vi "setFont.vi"(8 "Error In":errorcluster, 9 "className (\"QWidget\")":string="QWidget", 10 "font":refnum<class "QFont.lvclass">, 11 "LQWidgetEngine In":refnum<class "LQWidgetEngine.lvclass">) -> (0 "Error Out":errorcluster, 3 "LQWidgetEngine Out":refnum<class "LQWidgetEngine.lvclass">)   [LabVIEW 2014, in "LQWidgetEngine.lvclass"]
doc: "LabVIEW-specific documentation is not yet available. See <b>https://doc.qt.io/qt-5/qapplication.html#setFont</b>"
uses:
  LQWidgetEngine.lvclass
  Qt GUI/QFont/QFont.lvclass
  LQ Core/LQIdentity/LQIdentity.lvclass/LQIdentity.ctl
  LQ Core/LQSerialData/LQSerialData.lvclass/LQSerialData.ctl
  LQ Core/LQ Core.lvlib
  LQ Core/LQIdentity/LQIdentity.lvclass
  LQ Core/LQSerialData/LQSerialData.lvclass
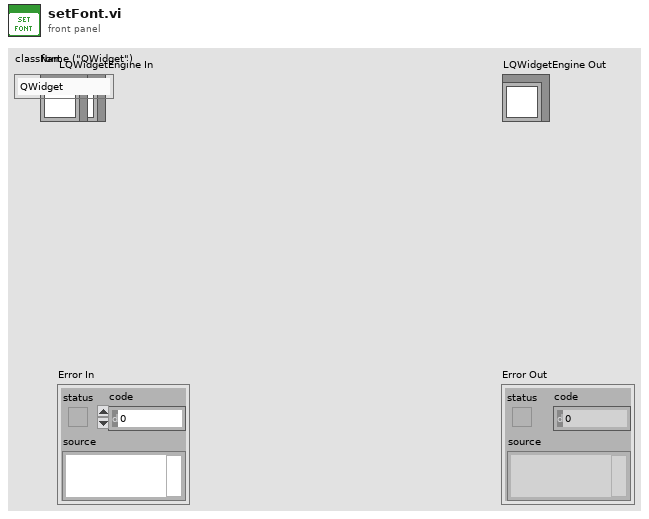
[diagram p1: front panel]
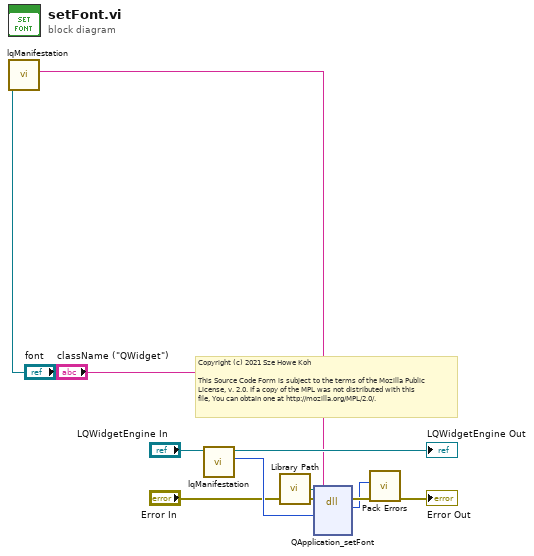
[diagram p0: block diagram]
diagram:
  # "Copyright (c) 2021 Sze Howe Koh\n\nThis Source Code Form is subject to the terms of the Mozilla Public\nLicense, v. 2.0. If a copy of the MPL was not distributed with this\nfile, You can obtain one at http://mozilla.org/MPL/2.0/."
  n1 = call "lqManifestation.vi"("LQSerialData in"="font") -> ("Manifestation"=w2:string)  [unwired: 9 in, 1 out]
  n2 = call "lqManifestation.vi"("LQIdentity in"="LQWidgetEngine In") -> ("Manifestation"=w8:u64, "LQIdentity out"=→"LQWidgetEngine Out":refnum<class "LQWidgetEngine.lvclass">)  [unwired: 9 in]
  n3 = call "Library Path.vi"() -> ("Library Path"=w9:path)
  n4 = dll-call lib="?" fn="QApplication_setFont"(path in=w9, error in="Error In", "_instance"=w8, "font"=w2, "className"="className (\"QWidget\")") -> (error out=w6:errorcluster, w4:i32)  [unwired: 4 in, 1 out]
  n5 = call "Pack Errors.vi"("Error In"=w6, "Error Code"=w4) -> ("Error Out"=→"Error Out":errorcluster)  [unwired: 9 in]
